vi "FFT_and_FindPeak_for_OneToneChannel_20190910.vi"(5 "Now.Target":T8=enum."4", 7 "DynRange_Thresh":dbl, 9 "FP_User":T1={"#NoiseSums"=0, "Max_df"=0, "AvgAvg"=FALSE, "#Avg"=0, "AutoCenter"=FALSE, "Inclin"={"Vmin"=0.0, "Vmax"=0.0, "Angle_min"=0.0, "Angle_max"=0.0, "Offset"=0.0, "Pos_Neg"=FALSE}, "1"={"Cal_"={"Fine"=0.0, "Coarse_"=0.0}, "Beac"={"Fine"=0.0, "Coarse_"=0.0}, "Scale"={"Step4"=0.0, "Step5"=0.0, "Step6"=0.0, "Step7"=0.0}, "Offset"=0.0, "Scale_Noise"=0.0, "Scale_Step1"=0.0, "Scale_In_RT"=0.0, "ScaleMeas"=0.0, "FreqsToRemove"=[], "Width"=[0, 1633], "ScaleMeasEnum"=enum."1", "FilterEnab"=enum."None"}, "2"={"Cal_"={"Fine"=0.0, "Coarse_"=0.0}, "Beac"={"Fine"=0.0, "Coarse_"=0.0}, "Scale"={"Step4"=0.0, "Step5"=0.0, "Step6"=0.0, "Step7"=0.0}, "Offset"=0.0, "Scale_Noise"=0.0, "Scale_Step1"=0.0, "Scale_In_RT"=0.0, "ScaleMeas"=0.0, "FreqsToRemove"=[], "Width"=[0, 1633], "ScaleMeasEnum"=enum."1", "FilterEnab"=enum."None"}, "3"={"Cal_"={"Fine"=0.0, "Coarse_"=0.0}, "Beac"={"Fine"=0.0, "Coarse_"=0.0}, "Scale"={"Step4"=0.0, "Step5"=0.0, "Step6"=0.0, "Step7"=0.0}, "Offset"=0.0, "Scale_Noise"=0.0, "Scale_Step1"=0.0, "Scale_In_RT"=0.0, "ScaleMeas"=0.0, "FreqsToRemove"=[], "Width"=[0, 1633], "ScaleMeasEnum"=enum."1", "FilterEnab"=enum."None"}, "4"={"Cal_"={"Fine"=0.0, "Coarse_"=0.0}, "Beac"={"Fine"=0.0, "Coarse_"=0.0}, "Scale"={"Step4"=0.0, "Step5"=0.0, "Step6"=0.0, "Step7"=0.0}, "Offset"=0.0, "Scale_Noise"=0.0, "Scale_Step1"=0.0, "Scale_In_RT"=0.0, "ScaleMeas"=0.0, "FreqsToRemove"=[], "Width"=[0, 1633], "ScaleMeasEnum"=enum."1", "FilterEnab"=enum."None"}, "Target to Probe"=enum."1", "SNR_Thresh"=0.0, "Paths"={"CfgFile"=path "", "LogFolder"=path "", "LogFile"=path "", "NAS path"=path "", "ThreshFile"=path "", "RedunFolder"=path ""}, "Connex_Location"="", "SimulateFPGA"=FALSE, "Deadband"=0.0} {"Deadband" format="%#.0f"}, 10 "f":dbl, 11 "Tone In":T10={"Shift_"=0.0, "Peak_ToFPGA"=-24999462.633451957, "MaxValue"=0.0, "MaxIndex"=0, "Tone"={"PkLocTrak"=0.0, "PkLocDisp"=0.0, "df_"=0.0, "ZoomPwr"=[], "Phase"=0.0, "PhaseOld"=0.0, "AboveThresh?"=FALSE, "MaxI"=0.0, "MaxQ"=0.0, "median"=0.0, "ISpect"=[], "QSpect"=[], "DeltaPhase"=0.0}, "TimeDomainI"=[], "TimeDomainQ"=array[12500 elements], "PwrSpectrum"=[], "RunningAvgFreq"=0.0, "ISpectPos"=[], "ISpectNeg"=[], "QSpectPos"=[], "QSpectNeg"=[], "10Hz_PwrSpectr"=[], "SNR"=0.0, "AliasWarn"=FALSE, "10Hz_Peak"=[], "ISpect+-"=[], "QSpect+-"=[], "TimeStamp"=timestamp(0 s since 1904-01-01), "I_Index"=array[12500 elements], "Q_Index"=array[12500 elements], "10MHz"=FALSE} {"Tone"."median" format="%0.2f"; "Tone"."MaxQ" format="%0.2f"}) -> (0 "PkLocTrak":dbl, 2 "MaxIndex":i32, 3 "Tone Out":T10={"Shift_"=0.0, "Peak_ToFPGA"=-24999462.633451957, "MaxValue"=0.0, "MaxIndex"=0, "Tone"={"PkLocTrak"=0.0, "PkLocDisp"=0.0, "df_"=0.0, "ZoomPwr"=[], "Phase"=0.0, "PhaseOld"=0.0, "AboveThresh?"=FALSE, "MaxI"=0.0, "MaxQ"=0.0, "median"=0.0, "ISpect"=[], "QSpect"=[], "DeltaPhase"=0.0}, "TimeDomainI"=[], "TimeDomainQ"=array[12500 elements], "PwrSpectrum"=[], "RunningAvgFreq"=0.0, "ISpectPos"=[], "ISpectNeg"=[], "QSpectPos"=[], "QSpectNeg"=[], "10Hz_PwrSpectr"=[], "SNR"=0.0, "AliasWarn"=FALSE, "10Hz_Peak"=[], "ISpect+-"=[], "QSpect+-"=[], "TimeStamp"=timestamp(0 s since 1904-01-01), "I_Index"=array[12500 elements], "Q_Index"=array[12500 elements], "10MHz"=FALSE} {"Tone"."median" format="%0.2f"; "Tone"."MaxQ" format="%0.2f"}, 4 "Shift_":dbl, 6 "x > y?":bool)   [LabVIEW 2018]
doc: "Perform FFT on ONE tone; either Cal or Beacon"
uses:
  Controls/Clusts/ChannelToneData.ctl
  Controls/ToneInfoClust.ctl
  Controls/Enums/TargetNumber.ctl
  Controls/Clusts/FrontPanel_UserConfig.ctl
  Controls/Clusts/Inclinometer_User_Cfg.ctl
  Controls/Clusts/FP_UserTargetConfig.ctl
  Controls/Clusts/FreqShift.ctl
  Controls/Clusts/FPGA_Scale.ctl
  Controls/Enums/ScaleMeasure.ctl
  Controls/RadioButtons/FilterEnableRadio.ctl
  Controls/PathsCluster.ctl
panel:
  out "RMS":dbl
  out "min value":dbl
  out "max value":dbl
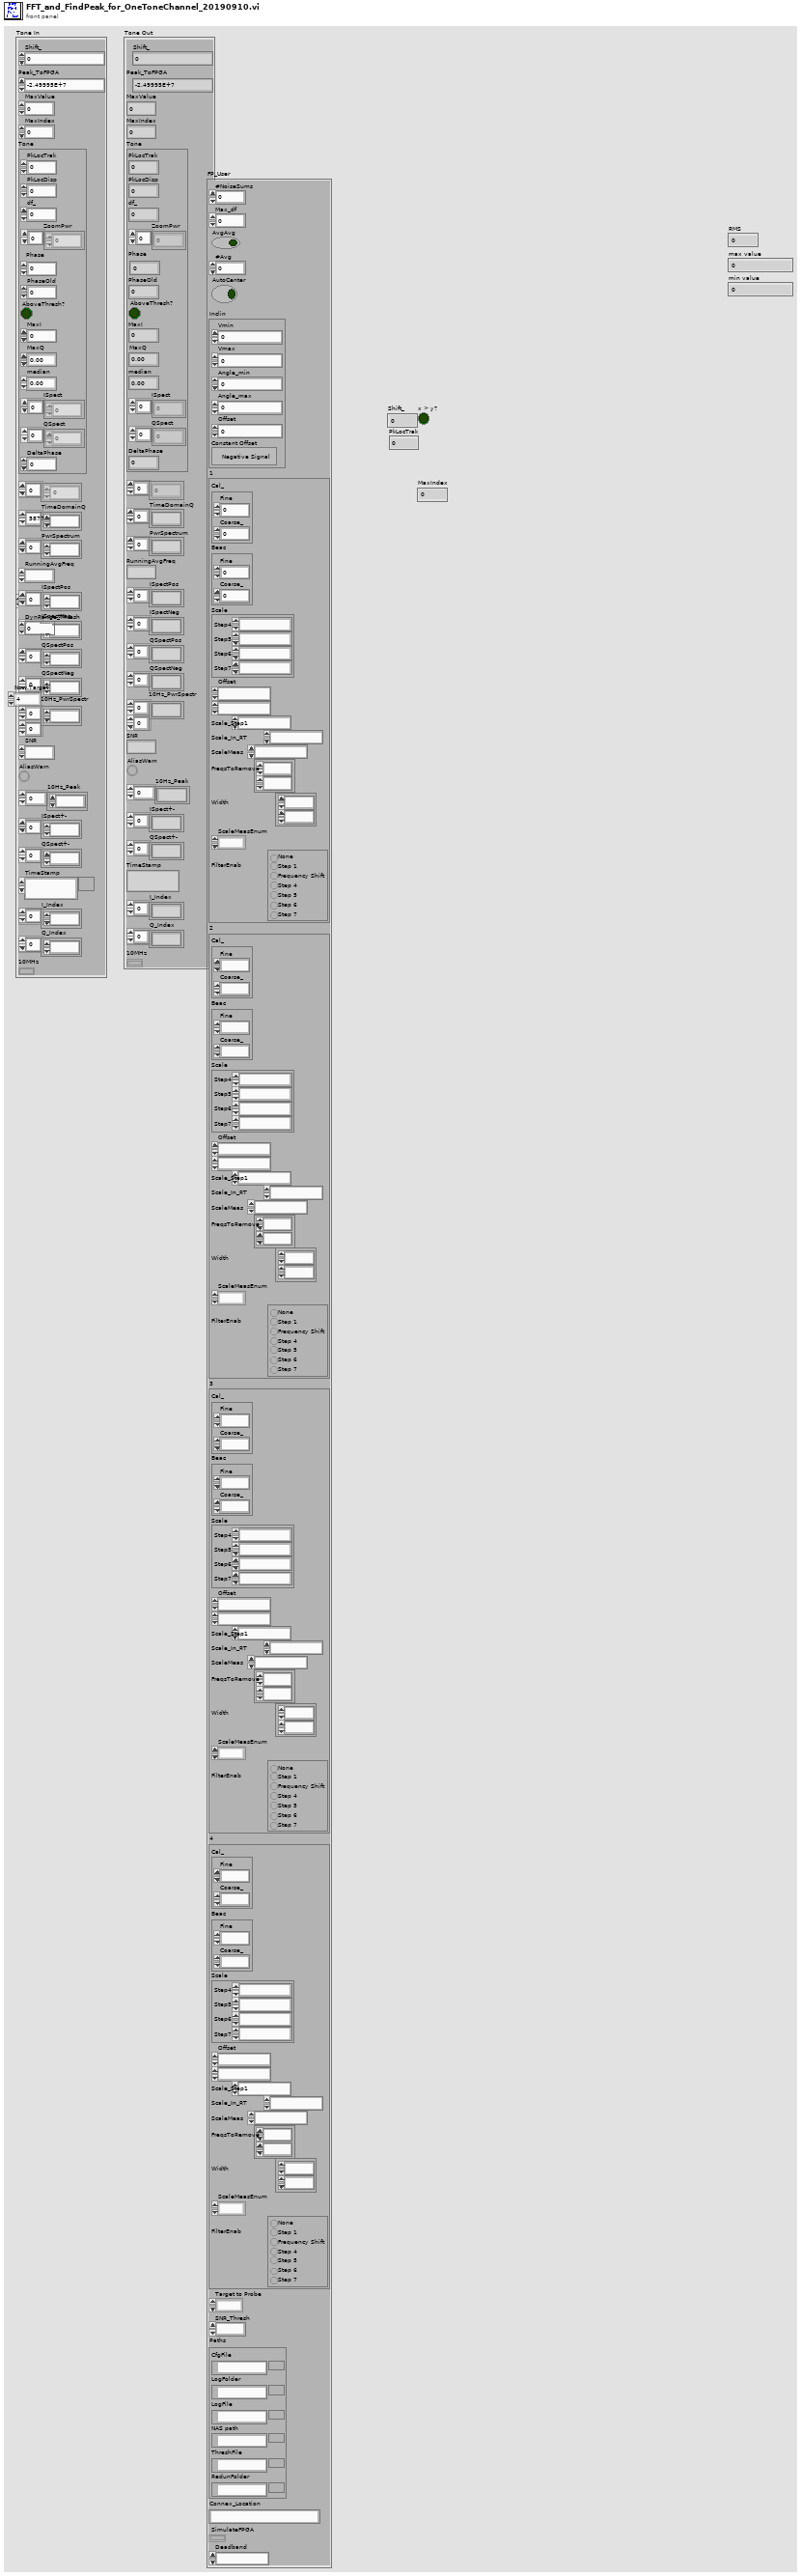
[diagram p1: front panel]
types:
  T1 = typedef "FrontPanel_UserConfig.ctl" = cluster{"#NoiseSums":u32, "Max_df":u32, "AvgAvg":bool, "#Avg":u16, "AutoCenter":bool, "Inclin":T2, "1":T3, "2":T3, "3":T3, "4":T3, "Target to Probe":T8, "SNR_Thresh":dbl, "Paths":T9, "Connex_Location":string, "SimulateFPGA":bool, "Deadband":dbl}
  T2 = typedef "Inclinometer_User_Cfg.ctl" = cluster{"Vmin":dbl, "Vmax":dbl, "Angle_min":dbl, "Angle_max":dbl, "Offset":dbl, "Pos_Neg":bool}
  T3 = typedef "FP_UserTargetConfig.ctl" = cluster{"Cal_":T4, "Beac":T4, "Scale":T5, "Offset":fxp<+/-,16,16>, "Scale_Noise":fxp<+/-,30,30>, "Scale_Step1":fxp<+/-,17,17>, "Scale_In_RT":ext, "ScaleMeas":fxp<+/-,16,1>, "FreqsToRemove":i32[], "Width":i32[], "ScaleMeasEnum":T6, "FilterEnab":T7}
  T4 = typedef "FreqShift.ctl" = cluster{"Fine":dbl, "Coarse_":dbl}
  T5 = typedef "FPGA_Scale.ctl" = cluster{"Step4":fxp<+/-,23,23>, "Step5":fxp<+/-,23,23>, "Step6":fxp<+/-,23,23>, "Step7":fxp<+/-,23,23>}
  T6 = typedef "ScaleMeasure.ctl" = enum16{"1", "10", "50", "42"}
  T7 = typedef "FilterEnableRadio.ctl" = enum32{"None", "Step 1", "Frequency Shift", "Step 4", "Step 5", "Step 6", "Step 7"}
  T8 = typedef "TargetNumber.ctl" = enum16{"1", "2", "3", "4"}
  T9 = typedef "PathsCluster.ctl" = cluster{"CfgFile":path, "LogFolder":path, "LogFile":path, "NAS path":path, "ThreshFile":path, "RedunFolder":path}
  T10 = typedef "ChannelToneData.ctl" = cluster{"Shift_":dbl, "Peak_ToFPGA":dbl, "MaxValue":dbl, "MaxIndex":i32, "Tone":T11, "TimeDomainI":ext[], "TimeDomainQ":ext[], "PwrSpectrum":dbl[], "RunningAvgFreq":dbl, "ISpectPos":dbl[], "ISpectNeg":dbl[], "QSpectPos":dbl[], "QSpectNeg":dbl[], "10Hz_PwrSpectr":dbl[][], "SNR":dbl, "AliasWarn":bool, "10Hz_Peak":dbl[], "ISpect+-":dbl[], "QSpect+-":dbl[], "TimeStamp":timestamp, "I_Index":ext[], "Q_Index":ext[], "10MHz":bool}
  T11 = typedef "ToneInfoClust.ctl" = cluster{"PkLocTrak":dbl, "PkLocDisp":dbl, "df_":dbl, "ZoomPwr":dbl[], "Phase":dbl, "PhaseOld":dbl, "AboveThresh?":bool, "MaxI":dbl, "MaxQ":dbl, "median":dbl, "ISpect":dbl[], "QSpect":dbl[], "DeltaPhase":dbl}
  T12 = typedef "ZoomSpectrumsClust.ctl" = cluster{"ZoomPowerSpectrum":dbl[], "MaxInPhase":dbl, "MaxQuadrature":dbl, "Phase":dbl, "ISpect":dbl[], "QSpect":dbl[]}
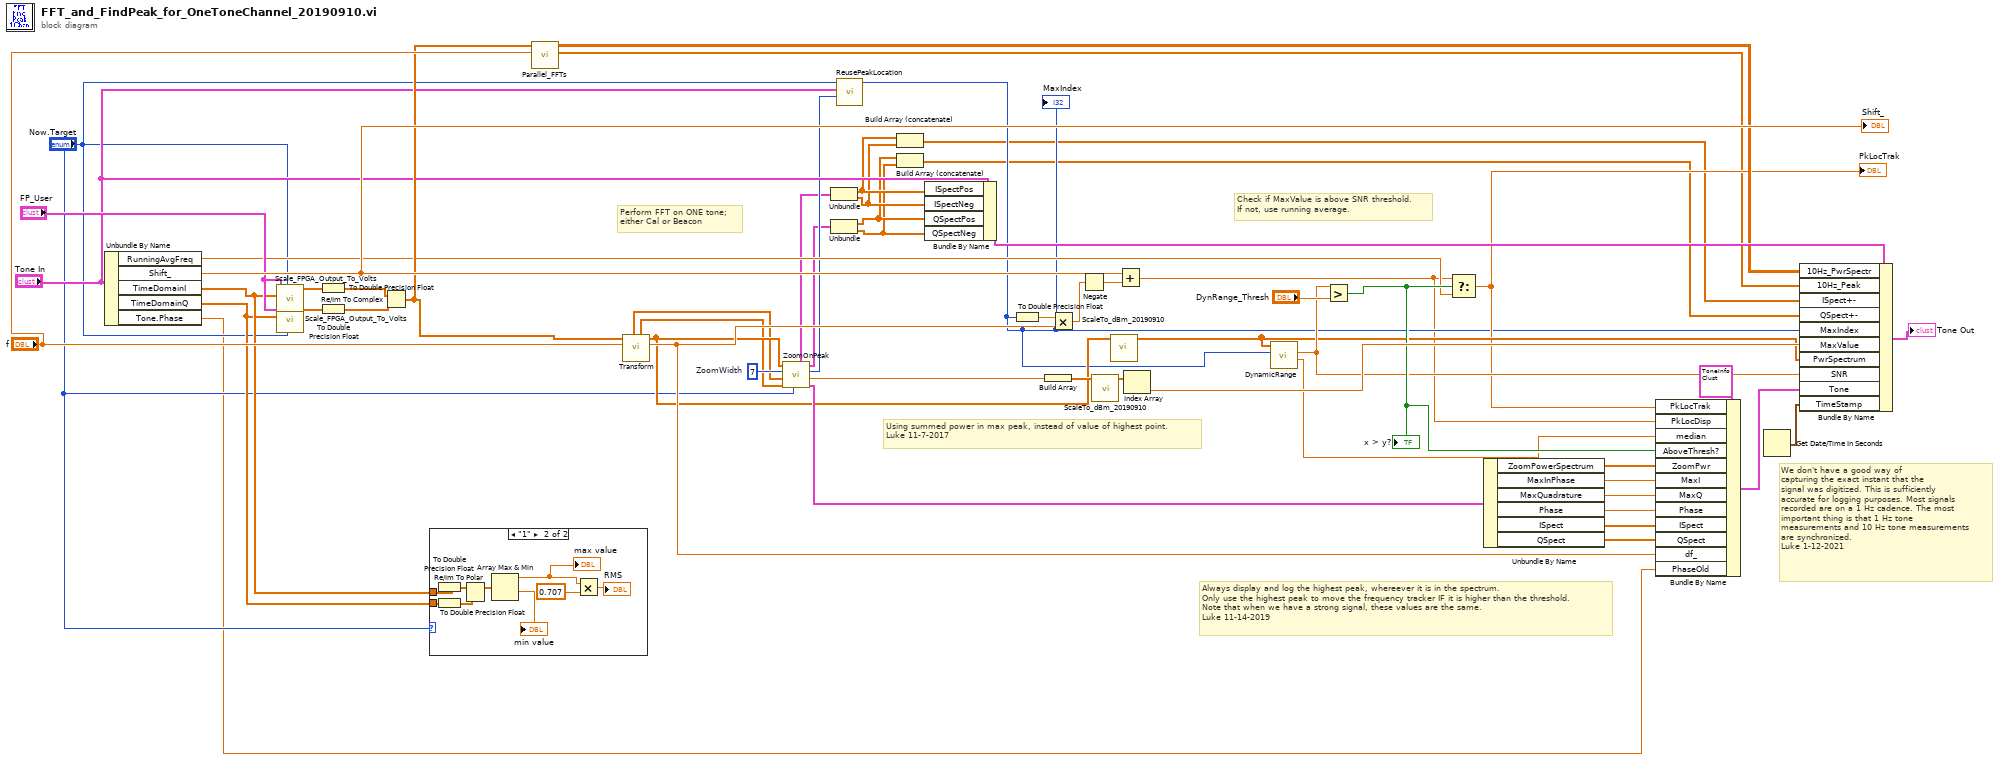
[diagram p0: block diagram]
diagram:
  w52 = 7  # ZoomWidth
  # "We don't have a good way of\ncapturing the exact instant that the\nsignal was digitized. This is sufficiently\naccurate for logging purposes. Most signals\nrecorded are on a 1 Hz cadence. The most\nimportant thing is that 1 Hz tone\nmeasurements and 10 Hz tone measurements\nare synchronized.\nLuke 1-12-2021"
  # "Always display and log the highest peak, whereever it is in the spectrum. \nOnly use the highest peak to move the frequency tracker IF it is higher than the threshold.\nNote that when we have a strong signal, these values are the same.\nLuke 11-14-2019"
  # "Check if MaxValue is above SNR threshold.\nIf not, use running average."
  # "Using summed power in max peak, instead of value of highest point.\nLuke 11-7-2017"
  # "Perform FFT on ONE tone;\neither Cal or Beacon"
  n1 = Unbundle By Name("Tone In") -> ("RunningAvgFreq"=w20:dbl, "Shift_"=w45:dbl, "TimeDomainI"=w26:ext[], "TimeDomainQ"=w25:ext[], "Tone.Phase"=w1:dbl)
  "Shift_" <- w45
  n2 = call "Scale_FPGA_Output_To_Volts.vi"("Chan#"="Now.Target", "FPGA_Data"=w26, "FP_User"="FP_User") -> ("Time Domain Volts"=w29:ext[])  [unwired: 7 in, 1 out]
  n3 = call "Scale_FPGA_Output_To_Volts.vi"("Chan#"="Now.Target", "FPGA_Data"=w25, "FP_User"="FP_User") -> ("Time Domain Volts"=w28:ext[])  [unwired: 7 in, 1 out]
  n4 = To Double Precision Float(number=w29) -> (double precision float=w23:dbl[])
  n5 = To Double Precision Float(number=w28) -> (double precision float=w22:dbl[])
  n6 = Re/Im To Complex(1:w22, 2:w23) -> (0:w24:cdb[])
  n7 = case shown="\"1\"" "Now.Target" {
    tunnel: w26 -> [_ w62]
    tunnel: w25 -> [_ w61]
    frame Default {
    }
    frame "1" {
      n8 = To Double Precision Float(number=w62) -> (double precision float=w60:dbl[])
      n9 = To Double Precision Float(number=w61) -> (double precision float=w59:dbl[])
      n10 = Re/Im To Polar(2:w59, 3:w60) -> (1:w58:dbl[])  [unwired: 1 out]
      n11 = Array Max & Min(array=w58) -> (max value=w65:dbl, min value=→"min value":dbl)  [unwired: 2 out]
      "max value" <- w65
      n12 = Multiply(x=w65, y=0.707) -> (x*y=→"RMS":dbl)
    }
  }
  n13 = call "Parallel_FFTs.vi"("SampleRate"="f", "Y"=w24) -> ("PeakValues"=w10:dbl[], "10 Hz FFTs"=w32:dbl[][])  [unwired: 8 in]
  n14 = call "Transform.vi"("SampleRate"="f", "TimeDomainIn"=w24) -> ("df (Hz)"=w57:dbl, "AmplitudeSpectrum"=w36:dbl[], "Quadrature"=w34:dbl[], "InPhase"=w35:dbl[])  [unwired: 4 in, 2 out]
  n15 = call "ZoomOnPeak.vi"("Now.Target"="Now.Target", "Quadrature spectrum in"=w34, "InPhase spectrum in"=w35, "ZoomWidth"=w52, "Power spectrum in"=w36) -> ("ZoomSpectrs"=w42:T12, "Power of Peak"=w43:dbl, "MaxIndex"=w18:i32, "ZoomQ"=w11:cluster{"ZoomQPos":dbl[], "ZoomQNeg":dbl[]}, "ZoomI"=w12:cluster{"ZoomIPos":dbl[], "ZoomINeg":dbl[]})  [unwired: 1 in, 1 out]
  n16 = Unbundle(w12) -> ("ZoomIPos"=w8:dbl[], "ZoomINeg"=w7:dbl[])
  n17 = Unbundle(w11) -> ("ZoomQPos"=w6:dbl[], "ZoomQNeg"=w5:dbl[])
  n18 = call "ReusePeakLocation.vi"("MaxIndex in"=w18, "Tone In"="Tone In", "Now.Target"="Now.Target") -> ("MaxIndex out"=w17:i32)  [unwired: 8 in]
  "MaxIndex" <- w17
  n19 = Build Array (concatenate)(w8, w7) -> (w4:dbl[])
  n20 = Build Array (concatenate)(w6, w5) -> (w3:dbl[])
  n21 = Bundle By Name(cluster="Tone In", "ISpectPos"=w8, "ISpectNeg"=w7, "QSpectPos"=w6, "QSpectNeg"=w5) -> (w46:T10)
  n22 = To Double Precision Float(number=w17) -> (double precision float=w37:dbl)
  n23 = Build Array(w43) -> (w48:dbl[])
  n24 = Multiply(x=w37, y=w57) -> (x*y=w54:dbl)
  n25 = Negate(x=w54) -> (-x=w51:dbl)
  n26 = call "ScaleTo_dBm_20190910.vi"("Power Spectrum In (Volts)"=w48) -> ("P (dBm)"=w50:dbl[])  [unwired: 10 in]
  n27 = call "ScaleTo_dBm_20190910.vi"("Power Spectrum In (Volts)"=w36) -> ("P (dBm)"=w30:dbl[])  [unwired: 10 in]
  n28 = Add(x=w45, y=w51) -> (x+y=w15:dbl)
  n29 = Index Array(array=w50) -> (element=w47:dbl)  [unwired: 1 in]
  n30 = call "DynamicRange.vi"("MaxIndex"=w17, "Power (dBm)"=w30) -> ("median"=w16:dbl, "DynamicRange"=w31:dbl)  [unwired: 8 in]
  n31 = Greater?(x=w31, y="DynRange_Thresh") -> (0:w44:bool)
  "x > y?" <- w44
  n32 = Select(t=w15, s=w44, f=w20) -> (s? t:f=w21:dbl)
  "PkLocTrak" <- w21
  n33 = Unbundle By Name(w42) -> ("ZoomPowerSpectrum"=w41:dbl[], "MaxInPhase"=w40:dbl, "MaxQuadrature"=w39:dbl, "Phase"=w38:dbl, "ISpect"=w14:dbl[], "QSpect"=w13:dbl[])
  n34 = Bundle By Name(cluster=T11 {"PkLocTrak"=0.0, "PkLocDisp"=0.0, "df_"=0.0, "ZoomPwr"=[], "Phase"=0.0, "PhaseOld"=0.0, "AboveThresh?"=FALSE, "MaxI"=0.0, "MaxQ"=0.0, "median"=0.0, "ISpect"=[], "QSpect"=[], "DeltaPhase"=0.0}, "PkLocTrak"=w21, "PkLocDisp"=w15, "median"=w16, "AboveThresh?"=w44, "ZoomPwr"=w41, "MaxI"=w40, "MaxQ"=w39, "Phase"=w38, "ISpect"=w14, "QSpect"=w13, "df_"=w57, "PhaseOld"=w1) -> (w55:T11)
  n35 = Get Date/Time In Seconds() -> (seconds since 1Jan1904=w2:timestamp)
  n36 = Bundle By Name(cluster=w46, "10Hz_PwrSpectr"=w32, "10Hz_Peak"=w10, "ISpect+-"=w4, "QSpect+-"=w3, "MaxIndex"=w17, "MaxValue"=w47, "PwrSpectrum"=w30, "SNR"=w31, "Tone"=w55, "TimeStamp"=w2) -> (→"Tone Out":T10)
